vi "NISE.Abort Session.vi"(8 "error in (no error)":errorcluster, 11 "SLSC Interface in":refnum<class "SLSC Interface.lvclass">) -> (0 "error out":errorcluster, 3 "SLSC Interface out":refnum<class "SLSC Interface.lvclass">)   [LabVIEW 2016, in "SLSC Interface.lvclass"]
uses:
  SLSC Interface.lvclass
  SLSC Interface.lvclass/SLSC Interface.ctl
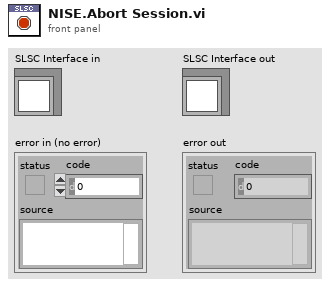
[diagram p1: front panel]
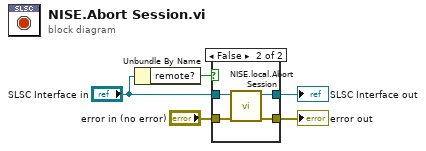
[diagram p0: block diagram]
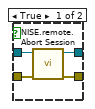
[diagram p2: hidden frame]
diagram:
  n1 = Unbundle By Name("SLSC Interface in") -> ("remote?"=w5:bool)
  n2 = case shown="False" w5 {
    tunnel: [w9 w13] -> w4
    tunnel: [w8 w12] -> w3
    tunnel: "error in (no error)" -> [w7 w11]
    tunnel: "SLSC Interface in" -> [w6 w10]
    frame True {
      n3 = call "NISE.remote.Abort Session.vi"("error in (no error)"=w7, "SLSC Remote in"=w6) -> ("error out"=w9:errorcluster, "SLSC Remote out"=w8:refnum<class "SLSC Interface.lvclass">)  [unwired: 8 in]
    }
    frame False {
      n4 = call "NISE.local.Abort Session.vi"("error in (no error)"=w11, "SLSC Local in"=w10) -> ("error out"=w13:errorcluster, "SLSC Local out"=w12:refnum<class "SLSC Interface.lvclass">)  [unwired: 8 in]
    }
  }
  "error out" <- w4
  "SLSC Interface out" <- w3
